vi "IMAQ Create.vi"(1 "Border Size":i32=3, 2 "Image Name":string="untitled", 5 "Image Type":u32(ring) items=["8 bits", "16 bits", "Float", "Complex", "RGB", "HSL"], 6 "error in (no error)":errorcluster) -> (0 "New Image":T1, 3 "error out":errorcluster)   [LabVIEW 2011]
doc: "Creates an image."
uses:
  IMAQ Image.ctl
  nivissvc.dll
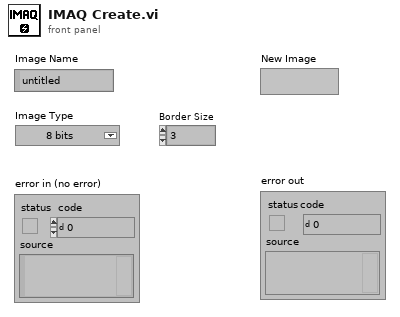
[diagram p1: front panel]
types:
  T1 = typedef "IMAQ Image.ctl" = cluster{string, u32}
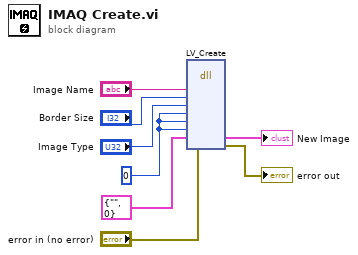
[diagram p0: block diagram]
diagram:
  w3 = 0
  n1 = dll-call lib="NIVisSvc.dll" fn="LV_Create"("name"="Image Name", "border"="Border Size", "imageType"="Image Type", "width"=w3, "height"=w3, "lock space"=w3, "New Image"=cluster{string, u32} {"", 0}, "error in (no error)"="error in (no error)") -> ("New Image"=→"New Image":cluster{string, u32}, "error in (no error)"=→"error out":errorcluster)  [unwired: 9 in, 3 out]
